vi "Untitled 4.vi"() -> ()   [LabVIEW 2019]
uses:
  <vilib>/rvi/Emulation/niFpgaGetClockAttributes.vi
  <vilib>/rvi/Emulation/niFpgaSctlEmulationGetInTimedLoop.vi
  <vilib>/rvi/Emulation/niFpgaEmulationReportErrorSimple.vi
  <vilib>/rvi/eio/common/nirviEmuTemplateMethod_errors.vi
  <vilib>/rvi/Emulation/niFpgaCriticalErrorInLSC.vi
  <vilib>/eio/EIONode/EIONode.xnode
panel:
  in  "reset":bool
  in  "stop":bool
  out "x+y":i16
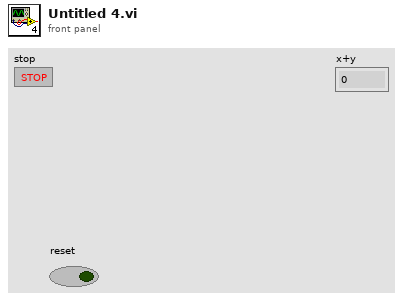
[diagram p1: front panel]
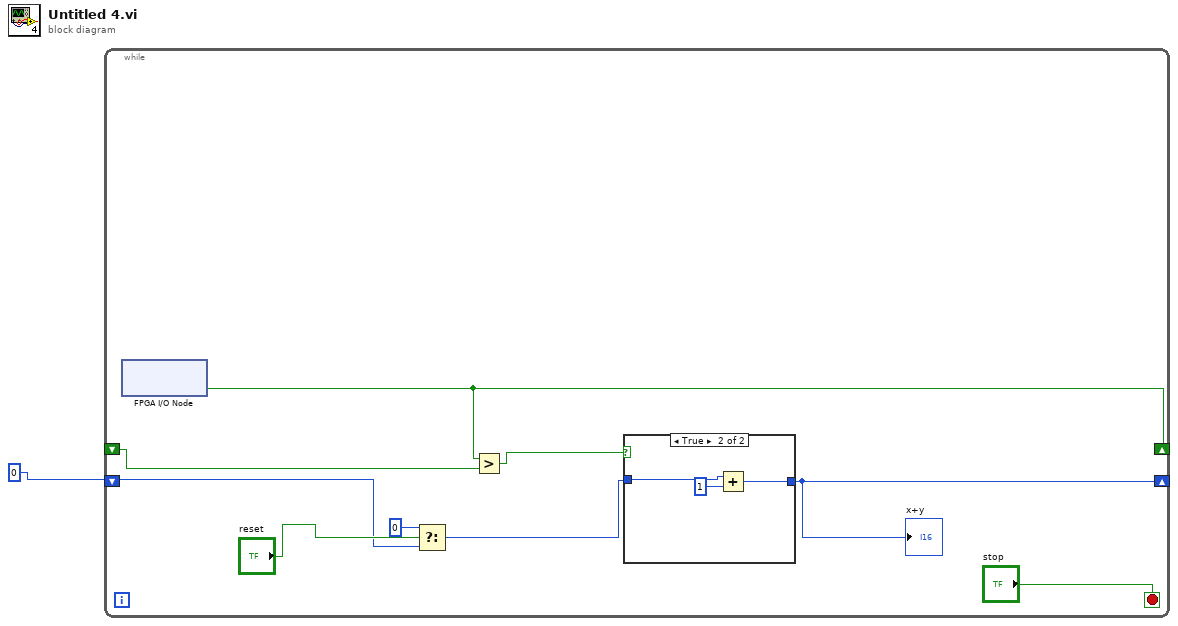
[diagram p0: block diagram]
diagram:
  n1 = while {
    shift-right: [w9] -> _
    shift-left: _ -> [w10]
    shift-right: [w7] -> _
    shift-left: i16 0 -> [w4]
    stop <- "stop" stop-if-true
    n2 = xnode "FPGA I/O Node"() -> ("Button0"=w9:bool)  [unwired: 1 in, 1 out]
    n3 = Select(t=i16 0, s="reset", f=w4) -> (s? t:f=w2:i16)
    n4 = Greater?(x=w9, y=w10) -> (0:w8:bool)
    n5 = case shown="True" w8 {
      tunnel: w2 -> [w11 w14]
      tunnel: [w11 w12] -> w7
      frame False {
      }
      frame True {
        n6 = Add(x=w14, y=i16 1) -> (x+y=w12:i16)
      }
    }
    "x+y" <- w7
  }
